vi "Write View Channel info.vi"(8 "error in":errorcluster, 10 "channel info":T1, 11 "channel in":refnum<class "StepNode.lvclass">) -> (0 "error out":errorcluster, 3 "channel out":refnum<class "StepNode.lvclass">)   [LabVIEW 2015]
doc: "Copyright 2017 National Instruments Corporation\n\nLicensed under the Apache License, Version 2.0 (the \"License\"); you may not use this file except in compliance with the License. You may obtain a copy of the License at http://www.apache.org/licenses/LICENSE-2.0\nUnless required by applicable law or agreed to in writing, software distributed under the License is distributed on an \"AS IS\" BASIS, WITHOUT WARRANTIES OR CONDITIONS OF ANY KIND, either express or implied. See the License for the specific language governing permissions and limitations under the License."
uses:
  StepNode.lvclass
  ChannelDisplayInfo.ctl
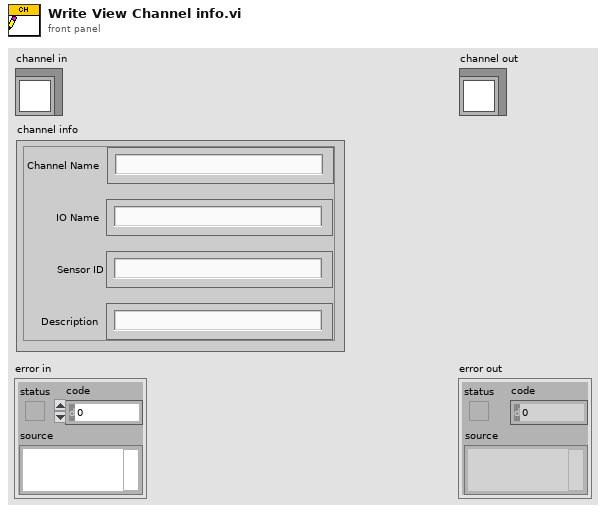
[diagram p1: front panel]
types:
  T1 = typedef "ChannelDisplayInfo.ctl" = cluster{"IO Name":string, "Sensor ID":string, "Channel Name":string, "Description ":string}
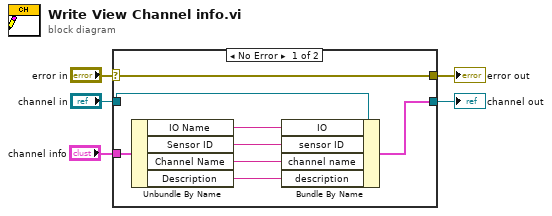
[diagram p0: block diagram]
diagram:
  n1 = case shown="No Error" "error in" {
    selector: "error in" -> [w13 w14]
    tunnel: [w13 w14] -> w4
    tunnel: [w7 w15] -> w2
    tunnel: "channel in" -> [w6 w15]
    tunnel: "channel info" -> [w8 _]
    frame No Error {
      n2 = Unbundle By Name(w8) -> ("IO Name"=w12:string, "Sensor ID"=w11:string, "Channel Name"=w10:string, "Description"=w9:string)
      n3 = Bundle By Name(cluster=w6, "IO"=w12, "sensor ID"=w11, "channel name"=w10, "description"=w9) -> (w7:cluster{})
    }
    frame Error {
    }
  }
  "error out" <- w4
  "channel out" <- w2
